vi "Test Broken test method.vi"(8 "error in (no error)":errorcluster, 11 "Test Case In":refnum<class "LUnit Comparison.lvclass">) -> (0 "error out":errorcluster, 3 "Test Case Out":refnum<class "LUnit Comparison.lvclass">)   [LabVIEW 2020, in "LUnit Comparison.lvclass"]
uses:
  LUnit Comparison.lvclass
  <vilib>/Astemes/LUnit/Test Case.lvclass
  C:/Program Files (x86)/National Instruments/LabVIEW 2020/vi.lib/Asteme/LUnit/Test Case.lvclass
  C:/Users/anton/Documents/GitHub/LUnit/sandbox/Benchmark/LUnit/Comparison Test/LUnit Comparison.lvclass
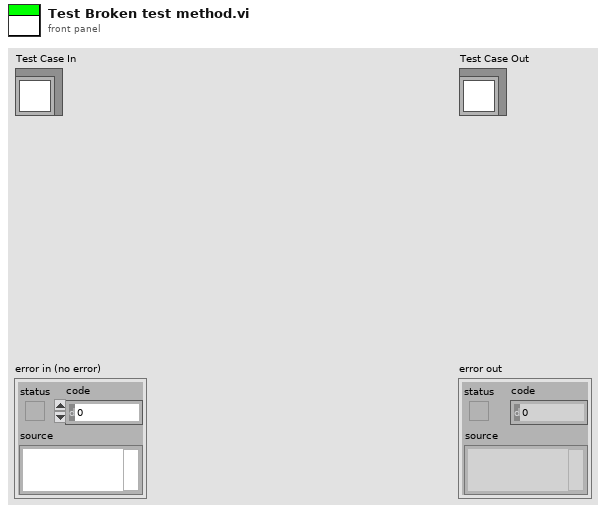
[diagram p1: front panel]
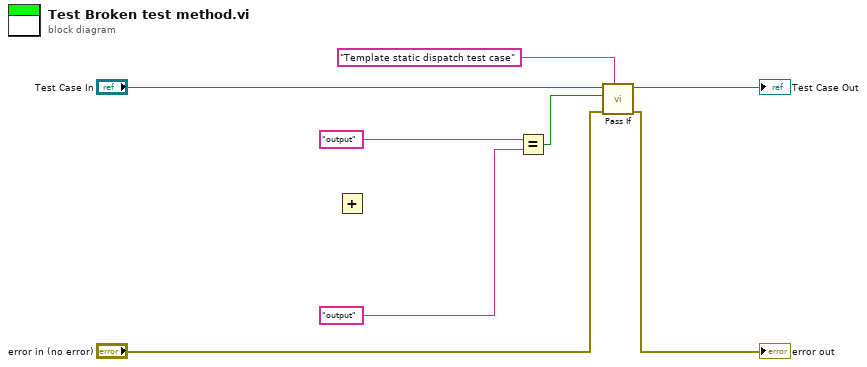
[diagram p0: block diagram]
diagram:
  n1 = Add() -> ()  [unwired: 2 in, 1 out]
  n2 = Equal?(x="output" ("Description"), y="output" ("Description")) -> (x = y?=w1:bool)
  n3 = call <vilib>:"Pass If.vi"("Description"="Template static dispatch test case", "error in (no error)"="error in (no error)", "Pass?"=w1, "LUnit Test Case In"="Test Case In") -> ("error out"=→"error out":errorcluster, "LUnit Test Case Out"=→"Test Case Out":refnum<class "LUnit Comparison.lvclass">)  [unwired: 6 in]
